vi "Configure Channels.vi"(8 "error in":errorcluster, 11 "DIO DAQmx PWM CFG in":refnum<class "CO DAQmx PWM CFG.lvclass">) -> (0 "error out":errorcluster, 3 "DIO DAQmx PWM CFG out":refnum<class "CO DAQmx PWM CFG.lvclass">)   [LabVIEW 2024, in "CO DAQmx PWM CFG.lvclass"]
uses:
  CO DAQmx PWM CFG.lvclass
  D:/git/HAL/HAL/Configurations/CFG Base/CFG Base.lvclass
  D:/git/HAL/HAL/Devices/DAQmx/DAQmx Base CFG/DAQmx Base CFG.lvclass
  DAQmx Base CFG/DAQmx Base CFG.lvclass/DAQmx Base CFG.ctl
  Configurations/CFG Base/CFG Base.lvclass/CFG Base.ctl
  f935c14f-6396-4c79-b521-c471996811ac.vi
  f935c14f-6396-4c79-b521-c471996811ac.vi/a4169a97-72fc-4003-a778-603cf20cafa0.vi
  <vilib>/JDP Science/JSONtext/Find Item.vi
  <vilib>/JDP Science/JSONtext/Next JSON Value.vi
  <vilib>/JDP Science/JSONtext/String Subset.vi
  <vilib>/JDP Science/JSONtext/Parsing/Advance past next JSON Value (inlined COPY).vi
  <vilib>/JDP Science/JSONtext/Parsing/Advance past whitespace.vi
  <vilib>/JDP Science/JSONtext/Parsing/Advance past String.vi
  <vilib>/JDP Science/JSONtext/Parsing/Advance past Number.vi
  <vilib>/JDP Science/JSONtext/Parsing/Advance past Line Ending.vi
  <vilib>/JDP Science/JSONtext/Parsing/Parse Full Path or Item Name.vi
  <vilib>/JDP Science/JSONtext/Parsing/Advance past Array.vi
  <vilib>/JDP Science/JSONtext/Parsing/Advance past Object.vi
  <vilib>/JDP Science/JSONtext/support/Error Cluster From Code.vi
  <vilib>/JDP Science/JSONtext/Offset/Find Item Locations by Path.vi
  <vilib>/JDP Science/JSONtext/JSON text to Variant.vi
  <vilib>/Utility/error.llb/Error Cluster From Error Code.vi
  <vilib>/DAQmx/create/channels.llb/DAQmx Create Channel (CO-Pulse Generation-Frequency).vi
  <vilib>/JDP Science/JSONtext/LVClass Serializer/JSONtext LVClass Serializer.lvclass
  CO DAQmx PWM CFG.lvclass/CO DAQmx PWM CFG.ctl
  DAQmx Base CFG/DAQmx Base CFG.lvclass
  Configurations/CFG Base/CFG Base.lvclass
  D:/git/HAL/HAL/Devices/DAQmx/DIO/CO DAQmx PWM CFG/CO DAQmx PWM CFG.lvclass
panel:
  out "Idle State":i32(ring)=10214 items=["High"=10192, "Low"=10214]
  out "Units":i32(ring)=10373 items=["Hz"=10373]
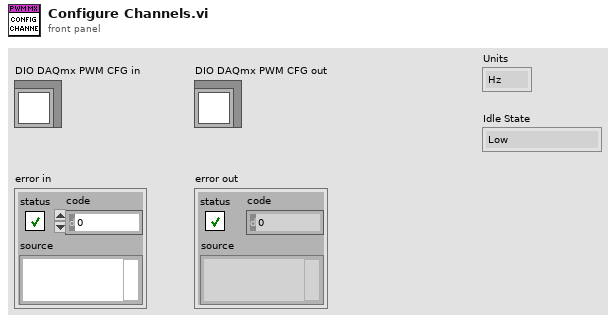
[diagram p1: front panel]
types:
  T1 = cluster{"Name":string, "Enabled":bool, "Duty Cycle":dbl, "Frequency":dbl, "Units":string, "Idle State":string, "Initial Delay":dbl}[]
  T2 = typedef "LVStringsAndValuesArrayTypeDef_I32.ctl" = cluster{"String":string, "Value":i32}[]
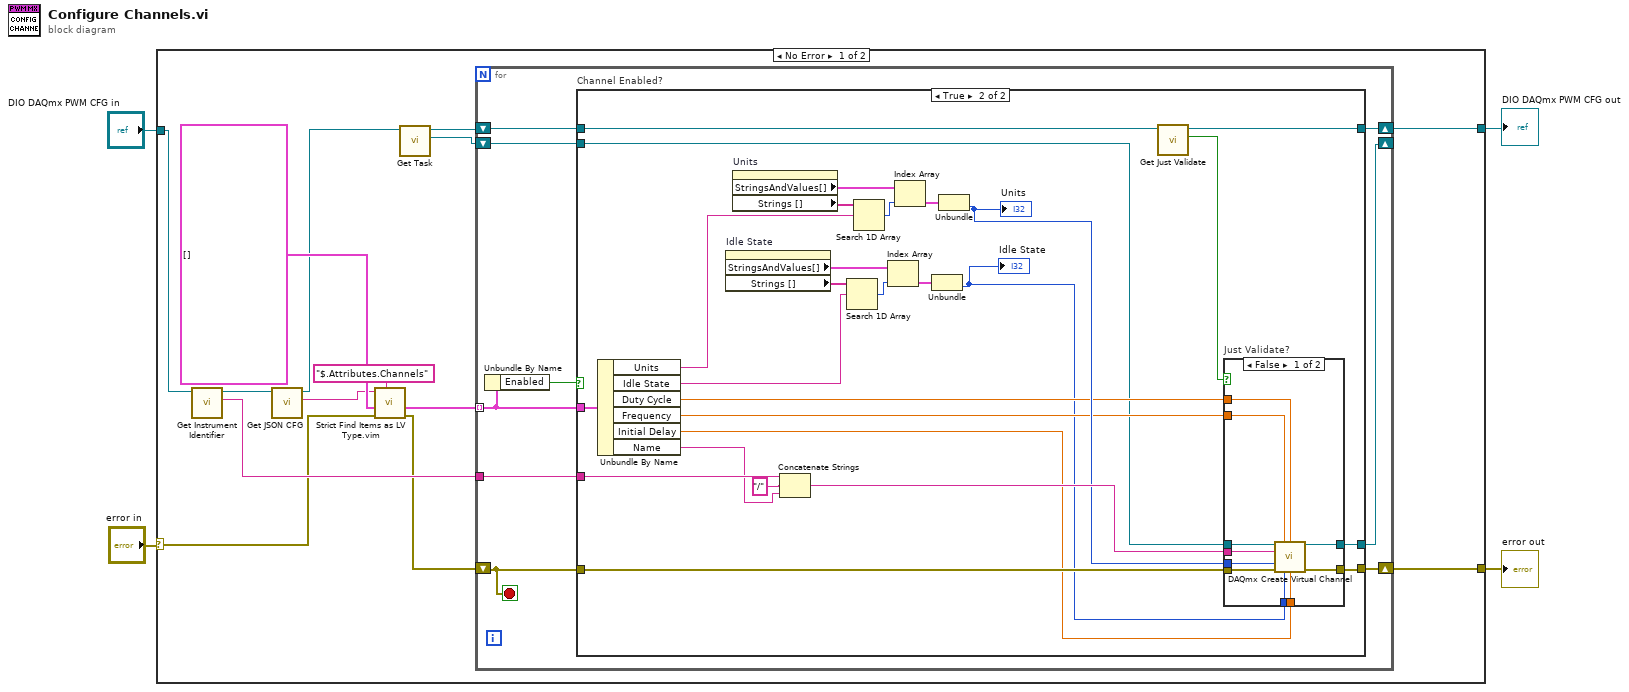
[diagram p0: block diagram]
diagram:
  n1 = case shown="No Error" "error in" {
    selector: "error in" -> [w5 w70]
    tunnel: "DIO DAQmx PWM CFG in" -> [w12 w71]
    tunnel: [w11 w70] -> w3
    tunnel: [w10 w71] -> w2
    frame No Error {
      n2 = call "Get Instrument Identifier.vi"("CFG Base in"=w12) -> ("Instrument Identifier"=w13:string, "CFG Base out"=w14:refnum<class "CO DAQmx PWM CFG.lvclass">)  [unwired: 9 in]
      n3 = call "Get JSON CFG.vi"("CFG Base in"=w14) -> ("<JSON>CFG"=w15:string, "CFG Base out"=w8:refnum<class "CO DAQmx PWM CFG.lvclass">)  [unwired: 9 in]
      n4 = call "Strict Find Items as LV Type.vim"("$Path or Item Name"="$.Attributes.Channels", "error in"=w5, "Data Type and Default Value"=T1 [], "<JSON>"=w15) -> ("error out"=w6:errorcluster, "Data out"=w17:T1)  [unwired: 5 in, 1 out]
      n5 = call "Get Task.vi"("DAQmx Base CFG in"=w8) -> ("Task"=w7:refnum<k21>, "DAQmx Base CFG out"=w9:refnum<class "CO DAQmx PWM CFG.lvclass">)  [unwired: 9 in]
      n6 = for {
        tunnel: w17 -> [w24] mode=indexing
        shift-right: [w27] -> w11
        shift-left: w6 -> [w26]
        tunnel: w13 -> [w25]
        shift-right: [w22] -> w10
        shift-left: w9 -> [w21]
        shift-right: [w20] -> _
        shift-left: w7 -> [w19]
        stop <- w26 stop-if-true
        n7 = Unbundle By Name(w24) -> ("Enabled"=w23:bool)
        n8 = case "Channel Enabled?" shown="True" w23 {
          tunnel: [w30 w36] -> w27
          tunnel: w26 -> [w30 w50]
          tunnel: w25 -> [_ w48]
          tunnel: w24 -> [_ w46]
          tunnel: [w29 w35] -> w22
          tunnel: w21 -> [w29 w32]
          tunnel: [w28 w33] -> w20
          tunnel: w19 -> [w28 w31]
          frame False {
          }
          frame True {
            n9 = Unbundle By Name(w46) -> ("Units"=w51:string, "Idle State"=w41:string, "Duty Cycle"=w40:dbl, "Frequency"=w39:dbl, "Initial Delay"=w37:dbl, "Name"=w47:string)
            n10 = property on="Idle State" class="Ring (strict)"() -> ("StringsAndValues[]"=w57:T2, "Strings []"=w43:string[])  [unwired: 2 in, 2 out]
            n11 = property on="Units" class="Ring (strict)"() -> ("StringsAndValues[]"=w53:T2, "Strings []"=w52:string[])  [unwired: 2 in, 2 out]
            n12 = Concatenate Strings(w48, "/" ("string"), w47) -> (w45:string)
            n13 = Search 1D Array(1D array=w43, element=w41) -> (index of element=w42:i32)  [unwired: 1 in]
            n14 = Search 1D Array(1D array=w52, element=w51) -> (index of element=w54:i32)  [unwired: 1 in]
            n15 = Index Array(array=w57, index=w42) -> (element=w56:cluster{"String":string, "Value":i32})
            n16 = Index Array(array=w53, index=w54) -> (element=w55:cluster{"String":string, "Value":i32})
            n17 = Unbundle(w56) -> ("Value"=w38:i32)  [unwired: 1 out]
            "Idle State" <- w38
            n18 = Unbundle(w55) -> ("Value"=w44:i32)  [unwired: 1 out]
            "Units" <- w44
            n19 = call "Get Just Validate.vi"("CFG Base in"=w32) -> ("Just Validate"=w34:bool, "CFG Base out"=w35:refnum<class "CO DAQmx PWM CFG.lvclass">)  [unwired: 9 in]
            n20 = case "Just Validate?" shown="False" w34 {
              tunnel: w50 -> [w67 w69]
              tunnel: w45 -> [w66 _]
              tunnel: w44 -> [w65 _]
              tunnel: w40 -> [w64 _]
              tunnel: w39 -> [w63 _]
              tunnel: w38 -> [w62 _]
              tunnel: w37 -> [w61 _]
              tunnel: w31 -> [w60 w68]
              tunnel: [w59 w69] -> w36
              tunnel: [w58 w68] -> w33
              frame False {
                n21 = call-poly <vilib>:"DAQmx Create Virtual Channel.vi"("task in"=w60, "frequency"=w63, "duty cycle"=w64, "counter"=w66, "units"=w65, "error in"=w67, "idle state"=w62, "initial delay"=w61) -> ("task out"=w58:refnum<k21>, "error out"=w59:errorcluster)  [unwired: 6 in]
              }
              frame True {
              }
            }
          }
        }
      }
    }
    frame Error {
    }
  }
  "error out" <- w3
  "DIO DAQmx PWM CFG out" <- w2
